vi "Radau5_Init from Cluster.vi"(8 "error in (no error)":errorcluster, 9 "Radau5 Parameters":T1={"initial time"=0.0, "final time"=10.0, "Absolute Tolerance"=[], "Relative Tolerance"=[], "minimum time step"=1e-08, "maximum time step"=1.0, "initial time step"=0.01} {"initial time step" min=0.0; "maximum time step" min=0.0; "minimum time step" min=0.0}, 10 "Initial Value Y'":dbl[](array[numeric]), 11 "Initial Value Y":dbl[](array[numeric])) -> (3 "Simulation Data":T2 {"Absolute tolerance" format="%.1e"; "Relative tolerance" format="%.1e"; "Output of T" format="%.1e"; "proposed step size" format="%.1e"; "min step size" format="%.1e"; "max step size" format="%.1e"; "final time" format="%.1e"; "step size" format="%.1e"; "initial time" format="%.1e"})   [LabVIEW 2020, in "NI_DAE.lvlib"]
doc: "<B>init from cluster</B> initialize the <B>simulation data</B> cluster from <B>initial condition</B> and <B>simulation parameter</B>"
uses:
  <vilib>/gmath/NI_DAE.lvlib
  <vilib>/gmath/dae.llb/Radau5_Simulation Data.ctl
  <vilib>/gmath/dae.llb/Radau5_Diag Eval Stage.ctl
  <vilib>/gmath/dae.llb/Radau5_Parameters.ctl
panel:
  in  "Simulation Data Type":T2 {"Absolute tolerance" format="%.1e"; "Relative tolerance" format="%.1e"; "Output of T" format="%.1e"; "proposed step size" format="%.1e"; "min step size" format="%.1e"; "max step size" format="%.1e"; "final time" format="%.1e"; "step size" format="%.1e"; "initial time" format="%.1e"}
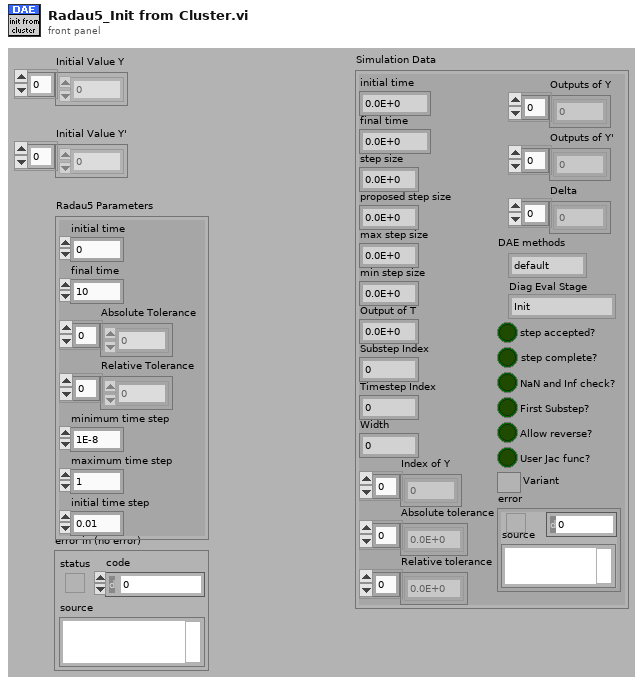
[diagram p1: front panel]
types:
  T1 = typedef "NI_DAE.lvlib/Radau5_Parameters.ctl" = cluster{"initial time":dbl, "final time":dbl, "Absolute Tolerance":dbl[], "Relative Tolerance":dbl[], "minimum time step":dbl, "maximum time step":dbl, "initial time step":dbl}
  T2 = typedef "NI_DAE.lvlib/Radau5_Simulation Data.ctl" = cluster{"initial time":dbl, "final time":dbl, "step size":dbl, "proposed step size":dbl, "max step size":dbl, "min step size":dbl, "Output of T":dbl, "Substep Index":i32, "Timestep Index":i32, "Width":i32, "Absolute tolerance":dbl[], "Relative tolerance":dbl[], "Outputs of Y":dbl[], "Outputs of Y'":dbl[], "Delta":dbl[], "DAE methods":enum16{"default", "Radau IIA"}, "Diag Eval Stage":T3, "step accepted?":bool, "step complete?":bool, "NaN and Inf check?":bool, "First Substep?":bool, "Allow reverse?":bool, "error":errorcluster, "User Jac func?":bool, "Variant":variant, "Index of Y":i8[]}
  T3 = typedef "NI_DAE.lvlib/Radau5_Diag Eval Stage.ctl" = enum16{"Init", "Running", "Final", "End"}
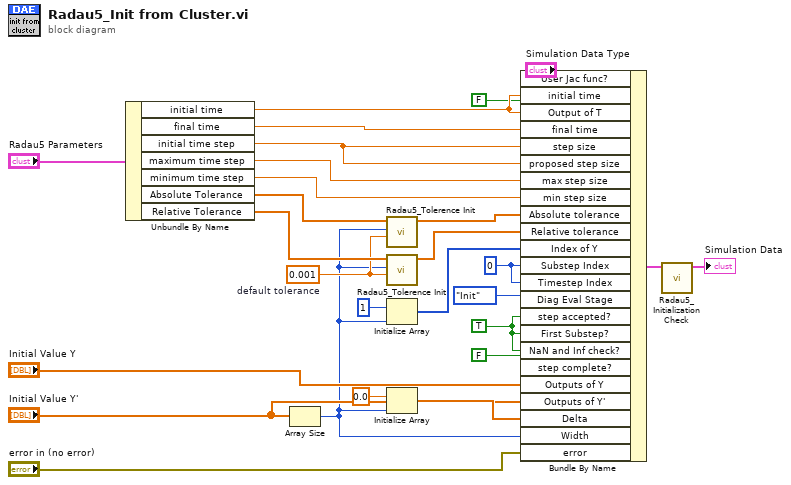
[diagram p0: block diagram]
diagram:
  w2 = 0.001  # default tolerance
  w16 = 0 ("Substep Index")
  w17 = TRUE ("step accepted?")
  n1 = Unbundle By Name("Radau5 Parameters") -> ("initial time"=w12:dbl, "final time"=w11:dbl, "initial time step"=w9:dbl, "maximum time step"=w8:dbl, "minimum time step"=w7:dbl, "Absolute Tolerance"=w6:dbl[], "Relative Tolerance"=w4:dbl[])
  n2 = Array Size(array="Initial Value Y'") -> (size(s)=w1:i32)
  n3 = call <vilib>:"Radau5_Tolerence Init.vi"("default tolerance"=w2, "width"=w1, "Tolerance input"=w6) -> ("Tolerance output"=w5:dbl[])  [unwired: 8 in]
  n4 = call <vilib>:"Radau5_Tolerence Init.vi"("default tolerance"=w2, "width"=w1, "Tolerance input"=w4) -> ("Tolerance output"=w3:dbl[])  [unwired: 8 in]
  n5 = Initialize Array(i8 1 ("element"), w1) -> (w14:i8[])
  n6 = Initialize Array(0.0 ("element"), w1) -> (w20:dbl[])
  n7 = Bundle By Name(cluster="Simulation Data Type", "User Jac func?"=FALSE, "initial time"=w12, "Output of T"=w12, "final time"=w11, "step size"=w9, "proposed step size"=w9, "max step size"=w8, "min step size"=w7, "Absolute tolerance"=w5, "Relative tolerance"=w3, "Index of Y"=w14, "Substep Index"=w16, "Timestep Index"=w16, "Diag Eval Stage"=Radau5_Diag_Eval_Stage."Init", "step accepted?"=w17, "First Substep?"=w17, "NaN and Inf check?"=w17, "step complete?"=FALSE ("step accepted?"), "Outputs of Y"="Initial Value Y", "Outputs of Y'"="Initial Value Y'", "Delta"=w20, "Width"=w1, "error"="error in (no error)") -> (w25:T2)
  n8 = call <vilib>:"Radau5_Initialization Check.vi"("Simulation data"=w25) -> ("Simulation data out"=→"Simulation Data":T2)  [unwired: 10 in]
